vi "All SubFunctions 6.vi"(4 "מק\"ט המכלל":string, 5 "מספר סידורי":string, 7 "מפעיל":string="ANS", 8 "error":errorcluster, 11 "Path for Log":path) -> (0 "error IO":errorcluster)   [LabVIEW 2015]
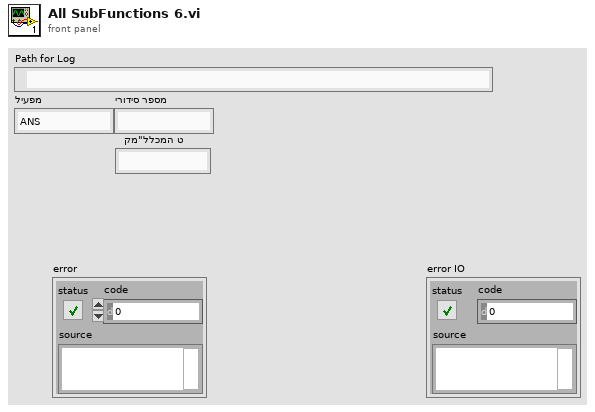
[diagram p1: front panel]
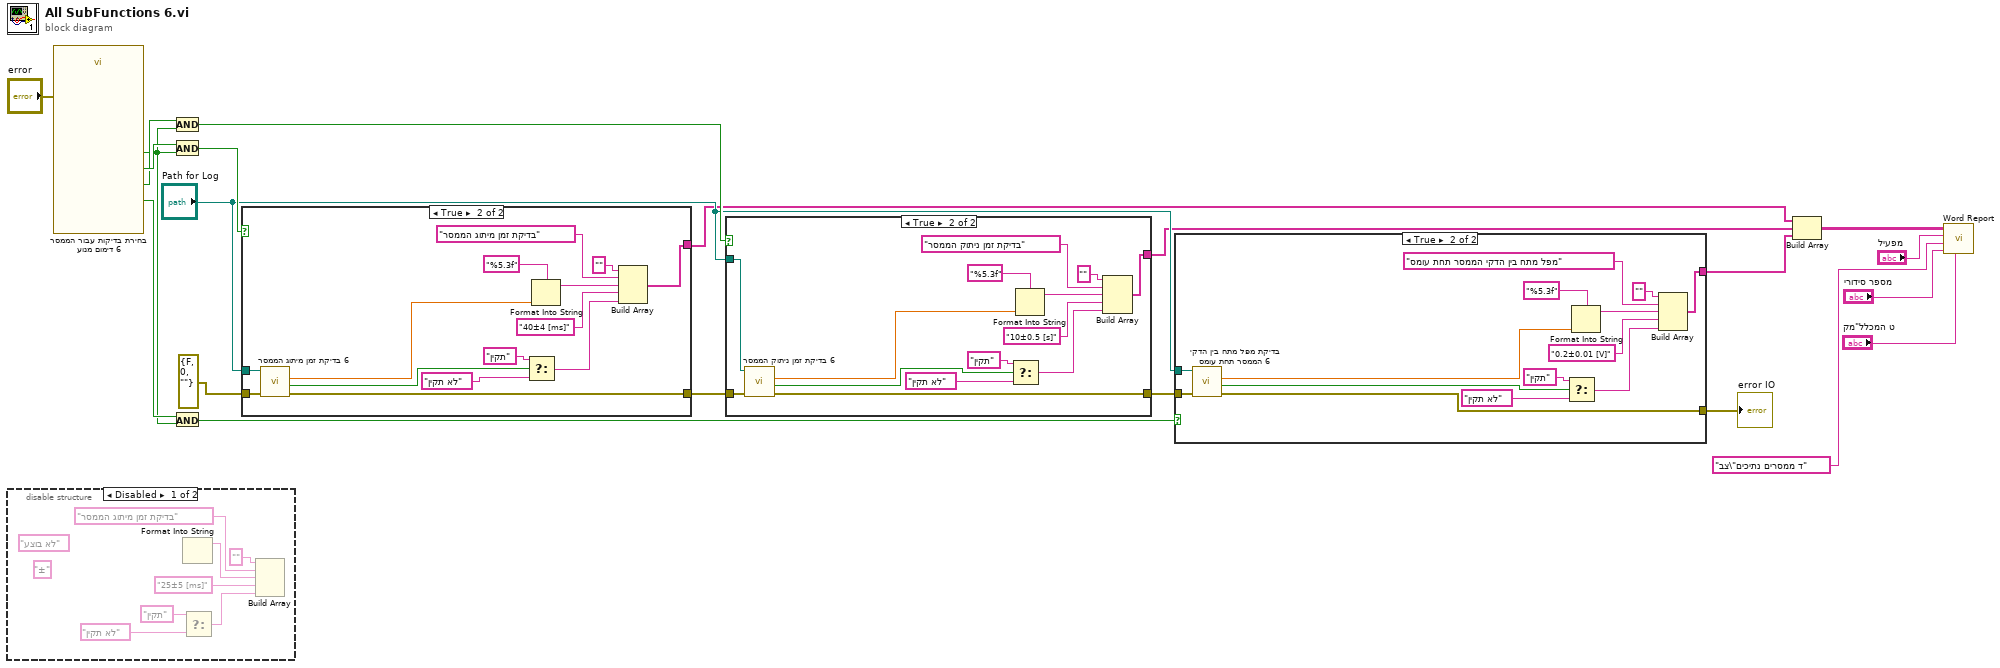
[diagram p0: block diagram]
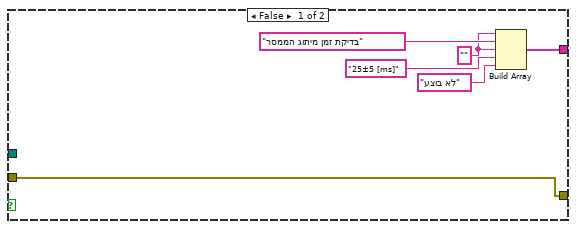
[diagram p3: hidden frame]
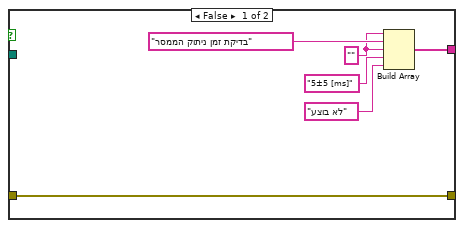
[diagram p4: hidden frame]
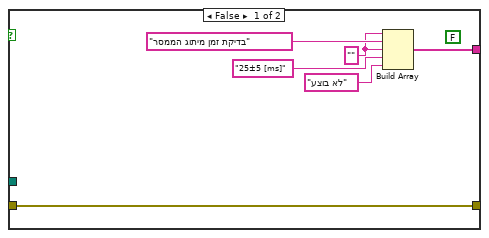
[diagram p5: hidden frame]
diagram:
  n1 = disable-structure shown="Disabled" {
    frame Disabled {
      (unwired) "±"
      (unwired) "לא בוצע"
      n2 = Format Into String() -> (resulting string=w26:string)  [unwired: 4 in, 1 out]
      n3 = Select(t="תקין", f="לא תקין") -> (s? t:f=w28:string)  [unwired: 1 in]
      n4 = Build Array("" ("element"), "בדיקת זמן מיתוג הממסר" ("element"), w26, "25±5 [ms]" ("element"), w28) -> ()  [unwired: 1 out]
    }
    frame Enabled {
    }
  }
  n5 = call "בחירת בדיקות עבור הממסר דימום מנוע 6.vi"("error in (no error)"="error") -> ("בדיקת מפל מתח בין דקי הממסר תחת עומס"=w13:bool, "בדיקת זמן ניתוק הממסר"=w15:bool, "בדיקת זמן מיתוג הממסר"=w17:bool, "OK"=w11:bool)  [unwired: 13 in, 2 out]
  n6 = And(x=w15, y=w11) -> (x .and. y?=w14:bool)
  n7 = And(x=w17, y=w11) -> (x .and. y?=w16:bool)
  n8 = And(x=w13, y=w11) -> (x .and. y?=w12:bool)
  n9 = case shown="True" w16 {
    tunnel: [w29 w48] -> w19
    tunnel: "Path for Log" -> [_ w47]
    tunnel: [w30 w37] -> w8
    tunnel: errorcluster {"status"=FALSE, "code"=0, "source"=""} ("error out") -> [w29 w35]
    frame False {
      w32 = "" ("element")
      (unwired) FALSE ("resultUserPrompt")
      n10 = Build Array(w32, "בדיקת זמן מיתוג הממסר" ("element"), w32, "25±5 [ms]" ("element"), "לא בוצע") -> (w30:string[])
    }
    frame True {
      n11 = call "בדיקת זמן מיתוג הממסר 6.vi"("error"=w35, "Path for Log"=w47) -> ("error out"=w48:errorcluster, "בטוח כן/לא"=w39:bool, "בדיקת זמן מיתוג הממסר"=w38:dbl)  [unwired: 7 in]
      n12 = Select(t="תקין", s=w39, f="לא תקין") -> (s? t:f=w40:string)
      n13 = Format Into String(format string="%5.3f", w38) -> (resulting string=w42:string)  [unwired: 2 in, 1 out]
      n14 = Build Array("" ("element"), "בדיקת זמן מיתוג הממסר" ("element"), w42, "40±4 [ms]" ("element"), w40) -> (w37:string[])
    }
  }
  n15 = case shown="True" w14 {
    tunnel: w19 -> [w54 w68]
    tunnel: [w54 w67] -> w18
    tunnel: "Path for Log" -> [_ w66]
    tunnel: [w49 w56] -> w7
    frame False {
      w50 = "" ("element")
      n16 = Build Array(w50, "בדיקת זמן ניתוק הממסר" ("element"), w50, "5±5 [ms]" ("element"), "לא בוצע") -> (w49:string[])
    }
    frame True {
      n17 = call "בדיקת זמן ניתוק הממסר 6.vi"("error"=w68, "Path for Log"=w66) -> ("error out"=w67:errorcluster, "בטוח כן/לא"=w57:bool, "בדיקת זמן ניתוק הממסר"=w58:dbl)  [unwired: 7 in]
      n18 = Select(t="תקין", s=w57, f="לא תקין") -> (s? t:f=w59:string)
      n19 = Format Into String(format string="%5.3f", w58) -> (resulting string=w61:string)  [unwired: 2 in, 1 out]
      n20 = Build Array("" ("element"), "בדיקת זמן ניתוק הממסר" ("element"), w61, "10±0.5 [s]" ("element"), w59) -> (w56:string[])
    }
  }
  n21 = case shown="True" w12 {
    tunnel: [w74 w88] -> w20
    tunnel: w18 -> [w74 w87]
    tunnel: "Path for Log" -> [_ w86]
    tunnel: [w69 w76] -> w6
    frame False {
      w70 = "" ("element")
      n22 = Build Array(w70, "בדיקת זמן מיתוג הממסר" ("element"), w70, "25±5 [ms]" ("element"), "לא בוצע") -> (w69:string[])
    }
    frame True {
      n23 = call "בדיקת מפל מתח בין הדקי הממסר תחת עומס 6.vi"("error"=w87, "Path for Log"=w86) -> ("error IO"=w88:errorcluster, "בטווח כן/לא"=w77:bool, "מפל מתח בין דקי הממסר תחת עומס"=w78:dbl)  [unwired: 6 in, 1 out]
      n24 = Select(t="תקין", s=w77, f="לא תקין") -> (s? t:f=w79:string)
      n25 = Format Into String(format string="%5.3f", w78) -> (resulting string=w81:string)  [unwired: 2 in, 1 out]
      n26 = Build Array("" ("element"), "מפל מתח בין הדקי הממסר תחת עומס" ("element"), w81, "0.2±0.01 [V]" ("element"), w79) -> (w76:string[])
    }
  }
  "error IO" <- w20
  n27 = Build Array(w8, w7, w6) -> (w9:string[][])
  n28 = call "Word Report.vi"("מק\"ט המכלל"="מק\"ט המכלל", "מספר סידורי"="מספר סידורי", "שם הצב\"ד"="צב\"ד ממסרים נתיכים", "מפעיל"="מפעיל", "Array"=w9) -> ()  [unwired: 7 in]
